vi "applyInsertSpace.vi"(4 "deltaY":u16, 6 "deltaX":u16, 8 "error in (no error)":errorcluster, 10 "origin":T1, 11 "GObject in":refnum<class "GObject.lvclass">) -> (0 "error out":errorcluster, 3 "GObject out":refnum<class "GObject.lvclass">)   [LabVIEW 2023, in "TLC_Scripto.lvlib" / "GObject.lvclass"]
uses:
  GObject.lvclass
  Ctrls/point.ctl
  GObject.lvclass/GObject.ctl
  TLC_Scripto.lvlib
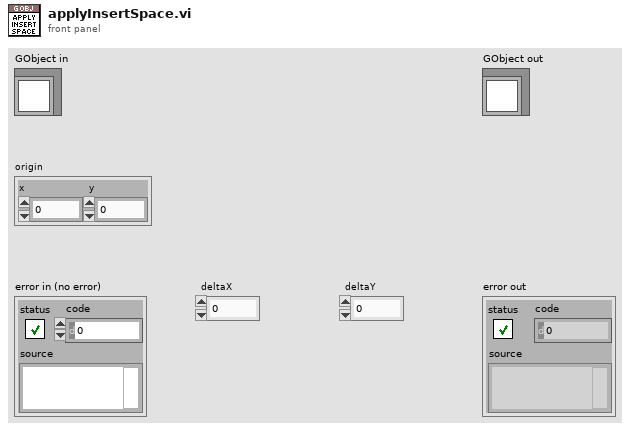
[diagram p1: front panel]
types:
  T1 = typedef "TLC_Scripto.lvlib/point.ctl" = cluster{"x":i32, "y":i32}
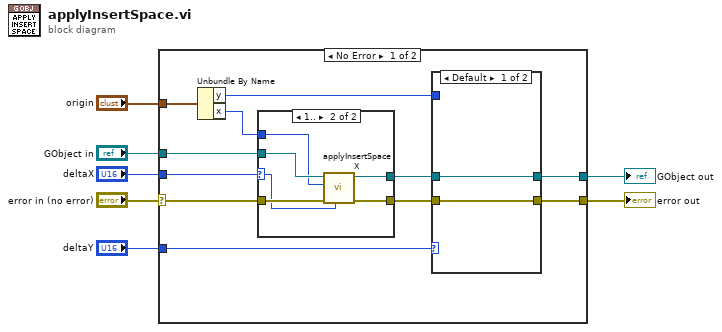
[diagram p0: block diagram]
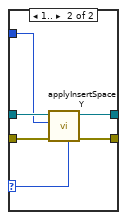
[diagram p2: hidden frame]
diagram:
  n1 = case shown="No Error" "error in (no error)" {
    selector: "error in (no error)" -> [w16 w36]
    tunnel: [w14 w36] -> w6
    tunnel: [w13 w35] -> w4
    tunnel: "GObject in" -> [w18 w35]
    tunnel: "deltaX" -> [w9 _]
    tunnel: "deltaY" -> [w8 _]
    tunnel: "origin" -> [w12 _]
    frame No Error {
      n2 = Unbundle By Name(w12) -> ("y"=w10:i32, "x"=w11:i32)
      n3 = case shown="1.." w9 {
        selector: w9 -> [_ w29]
        tunnel: w18 -> [w28 w34]
        tunnel: [w28 w33] -> w17
        tunnel: w16 -> [w27 w32]
        tunnel: [w27 w31] -> w15
        tunnel: w11 -> [_ w30]
        frame Default {
        }
        frame 1.. {
          n4 = call-dynamic "applyInsertSpaceX.vi"("deltaX"=w29, "error in (no error)"=w32, "originX"=w30, "GObject in"=w34) -> ("error out"=w31:errorcluster, "GObject out"=w33:refnum<class "GObject.lvclass">)  [unwired: 6 in]
        }
      }
      n5 = case shown="Default" w8 {
        selector: w8 -> [_ w21]
        tunnel: w17 -> [w20 w26]
        tunnel: w15 -> [w19 w25]
        tunnel: [w19 w24] -> w14
        tunnel: [w20 w23] -> w13
        tunnel: w10 -> [_ w22]
        frame Default {
        }
        frame 1.. {
          n6 = call-dynamic "applyInsertSpaceY.vi"("deltaY"=w21, "error in (no error)"=w25, "originY"=w22, "GObject in"=w26) -> ("error out"=w24:errorcluster, "GObject out"=w23:refnum<class "GObject.lvclass">)  [unwired: 6 in]
        }
      }
    }
    frame Error {
    }
  }
  "error out" <- w6
  "GObject out" <- w4
